vi "Place New Cricket.vi"(8 "error in (no error)":errorcluster, 9 "Packed refs":T1, 10 "Board Game in":refnum<class "Board Game.lvclass">, 11 "Cricket in":refnum<class "Cricket.lvclass">) -> (0 "error out":errorcluster, 1 "Rotation":enum16{"Clockwise", "CounterClockwise"}(ring), 3 "Cricket out":refnum<class "Cricket.lvclass">)   [LabVIEW 2021, in "Cricket.lvclass"]
uses:
  Cricket.lvclass
  C:/Users/poche/Programs/LabVIEW/imposible snake/GameEl_class/GameEl.lvclass
  Board Game_class/Board Game.lvclass
  Application/Packed Refs.ctl
  GameEl_class/private/Enum Direction.ctl
  LVApp/Modules/Sound Manager/Typedefs/Sound Effects.ctl
  Cricket.lvclass/Cricket.ctl
  GameEl_class/GameEl.lvclass/GameEl.ctl
  <vilib>/numeric/Random Number (Range) DBL.vi
  GameEl_class/GameEl.lvclass
  Application/Application.lvclass
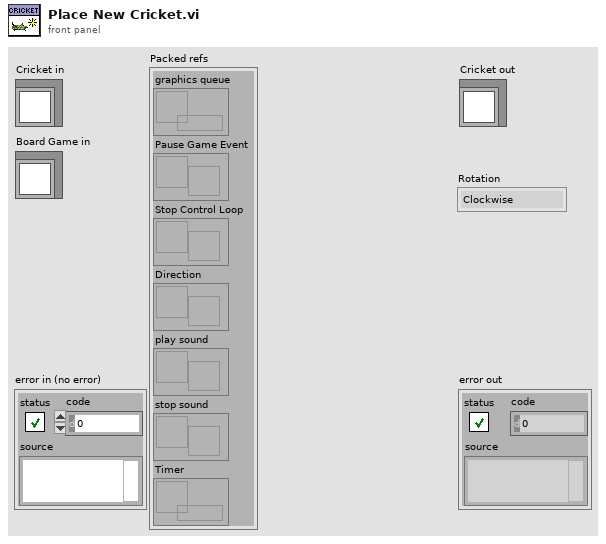
[diagram p1: front panel]
types:
  T1 = typedef "Application.lvclass/Packed Refs.ctl" = cluster{"graphics queue":refnum<queue>, "Pause Game Event":refnum<user-event>, "Stop Control Loop":refnum<user-event>, "Direction":refnum<notifier>, "play sound":refnum<user-event>, "stop sound":refnum<user-event>, "Timer":refnum<data-value>}
  T2 = typedef "Sound Effects.ctl" = enum16{"Bomb In", "Bomb Out", "Bomb Touched", "Game Over", "Victory", "Eat", "10 Fruits", "Eat2", "Eat3", "Eat4", "MaxShield", "Shield", "10p", "Grape In", "Grape Out", "20p", "30p", "40p", "50p", "60p", "70p", "80p", "90p", "100p", "All shields cracked", "Mouse In", "Mouse Out", "Mouse Eaten", "Grape Eaten", "States Recover", "Broken Shield", "Bonus", "Happy Time", "explode", "Game over musica", "Back Music", "Shield Catch", "Evil lough", "Cricket In", "Cricket eaten", "Lets Go", "Jump1", "Jump2", "Jump3", "Unstoppable", "Troll Music", "winner"}
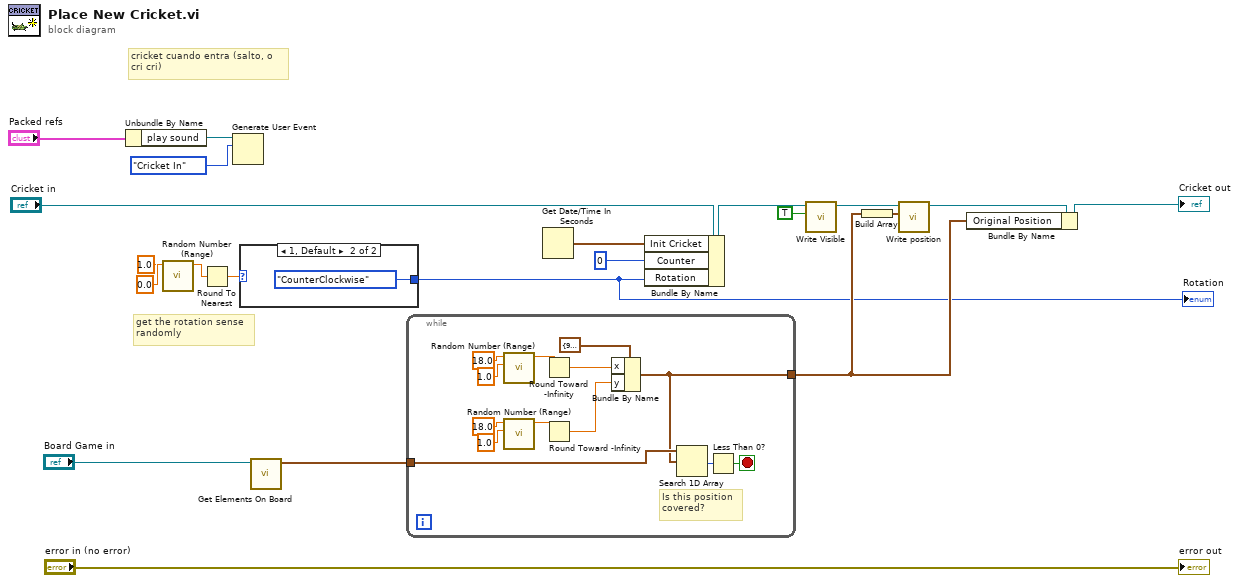
[diagram p0: block diagram]
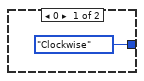
[diagram p2: hidden frame]
diagram:
  # "get the rotation sense \nrandomly"
  # "cricket cuando entra (salto, o \ncri cri)"
  n1 = Unbundle By Name("Packed refs") -> ("play sound"=w2:refnum<user-event>)
  n2 = call-poly <vilib>:"Random Number (Range).vi"("lower bound (0)"=1.0 ("High"), "upper bound (100)"=0.0 ("Low")) -> ("number"=w7:dbl)  [unwired: 9 in]
  n3 = Round To Nearest(number=w7) -> (nearest integer value=w6:dbl)
  n4 = Generate User Event(user event=w2, event data cluster=Sound_Effects."Cricket In" ("event data")) -> ()  [unwired: 2 in, 2 out]
  n5 = case shown="1, Default" w6 {
    tunnel: [enum16{"Clockwise", "CounterClockwise"}."Clockwise" ("Rotation") enum16{"Clockwise", "CounterClockwise"}."CounterClockwise" ("Rotation")] -> w3
    frame 0 {
    }
    frame 1, Default {
    }
  }
  "Rotation" <- w3
  n6 = call "Get Elements On Board.vi"("Board Game in"="Board Game in") -> ("position"=w15:cluster{"x":dbl, "y":dbl}[])  [unwired: 9 in, 1 out]
  n7 = while {
    tunnel: w15 -> [w36]
    tunnel: [w24] -> w4
    stop <- w34 stop-if-true
    # "Is this position \ncovered?"
    n8 = call-poly <vilib>:"Random Number (Range).vi"("lower bound (0)"=1.0 ("Low"), "upper bound (100)"=18.0 ("High")) -> ("number"=w28:dbl)  [unwired: 9 in]
    n9 = call-poly <vilib>:"Random Number (Range).vi"("lower bound (0)"=1.0 ("Low"), "upper bound (100)"=18.0 ("High")) -> ("number"=w25:dbl)  [unwired: 9 in]
    n10 = Round Toward -Infinity(1:w28) -> (0:w33:dbl)
    n11 = Round Toward -Infinity(1:w25) -> (0:w32:dbl)
    n12 = Bundle By Name(cluster=cluster{"x":dbl, "y":dbl} {"x"=9.0, "y"=20.0} ("position"), "x"=w33, "y"=w32) -> (w24:cluster{"x":dbl, "y":dbl})
    n13 = Search 1D Array(1D array=w36, element=w24) -> (index of element=w35:i32)  [unwired: 1 in]
    n14 = Less Than 0?(x=w35) -> (x < 0?=w34:bool)
  }
  n15 = Get Date/Time In Seconds() -> (seconds since 1Jan1904=w14:timestamp)
  n16 = Bundle By Name(cluster="Cricket in", "Init Cricket"=w14, "Counter"=u32 0, "Rotation"=w3) -> (w21:refnum<class "Cricket.lvclass">)
  n17 = call "Write Visible.vi"("Visible"=TRUE, "GameEl in"=w21) -> ("GameEl out"=w20:refnum<class "Cricket.lvclass">)  [unwired: 8 in, 1 out]
  n18 = Build Array(w4) -> (w18:cluster{"x":dbl, "y":dbl}[])
  n19 = call "Write position.vi"("position"=w18, "GameEl in"=w20) -> ("GameEl out"=w12:refnum<class "Cricket.lvclass">)  [unwired: 8 in, 1 out]
  n20 = Bundle By Name(cluster=w12, "Original Position"=w4) -> (→"Cricket out":refnum<class "Cricket.lvclass">)
  "error out" <- "error in (no error)"
